vi "Place on Cursor.vi"(8 "error in (no error)":errorcluster, 11 "name":string) -> (0 "error out":errorcluster, 3 "success?":bool)   [LabVIEW 2016]
doc: "(Wrapper VI)\n\nPlaces a palette object on the cursor so the object is ready to add to the front panel window or the block diagram window."
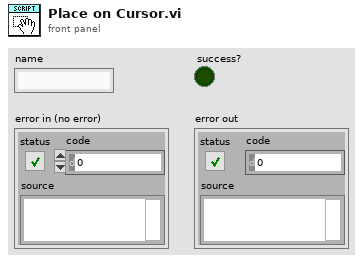
[diagram p1: front panel]
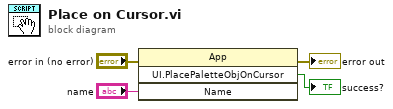
[diagram p0: block diagram]
diagram:
  n1 = invoke class="App" method="UI.PlacePaletteObjOnCursor"(error in="error in (no error)", "Name"="name") -> (error out=→"error out":errorcluster, "Drop Control Or Function"=→"success?":bool)  [unwired: 2 in, 2 out]
